vi "macro_MatrixHelper_CoerceSize.vi"   [LabVIEW 2019, in "Trajectory_Library.lvlib"]
uses:
  Trajectory_Library.lvlib
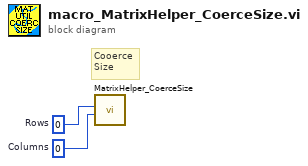
[diagram p0: block diagram]
diagram:
  w1 = 0  # Columns
  w2 = 0  # Rows
  # "Cooerce\nSize"
  n1 = call "MatrixHelper_CoerceSize.vi"("Columns"=w1, "Rows"=w2) -> ()  [unwired: 8 in, 2 out]
